vi "errorMsg.vi"(0 "error IO 2":errorcluster) -> (1 "error IO":errorcluster, 2 "T button?":bool)   [LabVIEW 2010]
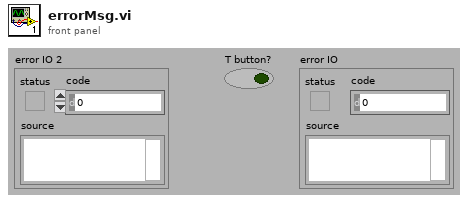
[diagram p1: front panel]
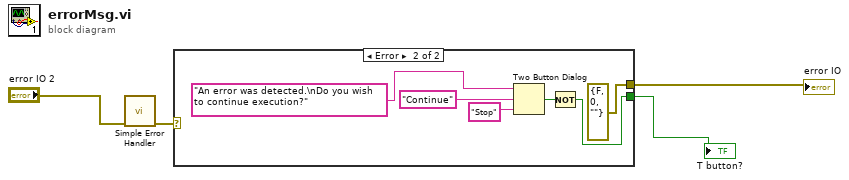
[diagram p0: block diagram]
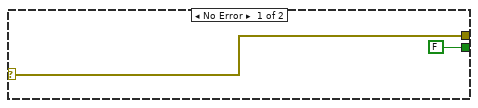
[diagram p2: hidden frame]
diagram:
  n1 = call <vilib>:"Simple Error Handler.vi"("error in (no error)"="error IO 2") -> ("error out"=w2:errorcluster)  [unwired: 1 in, 7 out]
  n2 = case shown="Error" w2 {
    selector: w2 -> [w6 _]
    tunnel: [w6 errorcluster {"status"=FALSE, "code"=0, "source"=""} ("error IO")] -> w4
    tunnel: [FALSE ("T button?") w8] -> w3
    frame No Error {
    }
    frame Error {
      n3 = Two Button Dialog(message="An error was detected.\nDo you wish to continue execution?", 1:"Stop" ("F button name (\"Cancel\")"), 2:"Continue" ("T button name (\"OK\")")) -> (T button?=w9:bool)
      n4 = Not(x=w9) -> (.not. x?=w8:bool)
    }
  }
  "error IO" <- w4
  "T button?" <- w3
